vi "Get Type.vi"(8 "error in (no error)":errorcluster, 11 "Plastic in":refnum<class "Plastic.lvclass">) -> (0 "error out":errorcluster, 2 "Item Type":T1, 3 "Plastic out":refnum<class "Plastic.lvclass">)   [LabVIEW 2020, in "Plastic.lvclass"]
uses:
  Plastic.lvclass
  Item/Item Type.ctl
  Item/Item.lvclass
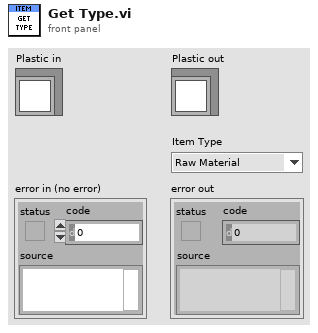
[diagram p1: front panel]
types:
  T1 = typedef "Item.lvclass/Item Type.ctl" = enum16{"Raw Material", "Component", "Module", "Product"}
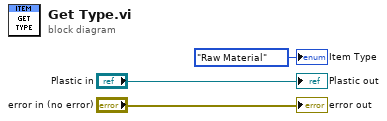
[diagram p0: block diagram]
diagram:
  "error out" <- "error in (no error)"
  "Plastic out" <- "Plastic in"
  "Item Type" <- Item_Type."Raw Material" ("Item Type")
